vi "监测项目写入.vi"(8 "error in (no error)":errorcluster caption="错误输入（无错误）", 10 "字符串与值":cluster{"字符串":string, "值":u16}[](array[cluster]), 11 "SingleStepTestV3 输入":refnum<class "SingleStepTestV2.lvclass">) -> (0 "error out":errorcluster caption="错误输出", 3 "SingleStepTestV3 输出":refnum<class "SingleStepTestV2.lvclass">)   [LabVIEW 2022 SP3, in "SingleStepTestV2.lvlib" / "SingleStepTestV2.lvclass"]
uses:
  SingleStepTestV2.lvclass
  SingleStepTestV2.lvclass/SingleStepTestV2.ctl
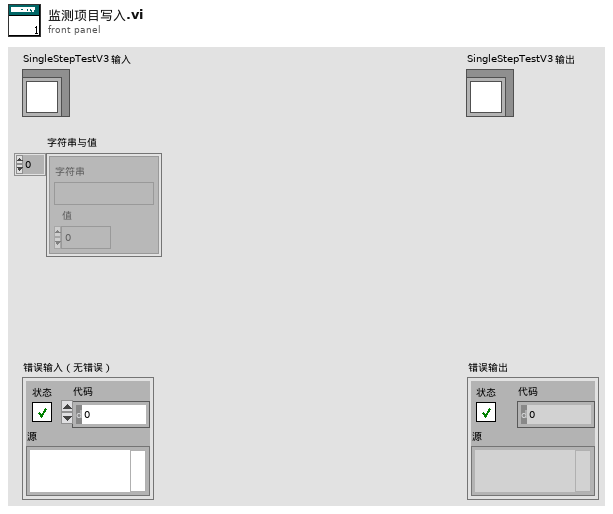
[diagram p1: front panel]
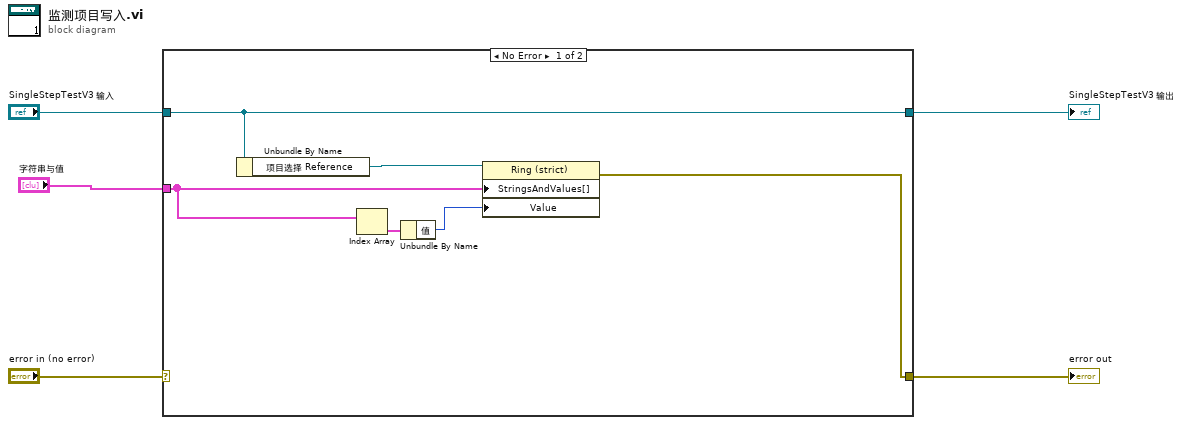
[diagram p0: block diagram]
diagram:
  n1 = case shown="No Error" "error in (no error)" {
    selector: "error in (no error)" -> [_ w13]
    tunnel: [w6 w13] -> w4
    tunnel: [w7 w12] -> w2
    tunnel: "SingleStepTestV3 输入" -> [w7 w12]
    tunnel: "字符串与值" -> [w11 _]
    frame No Error {
      n2 = Unbundle By Name(w7) -> ("项目选择 Reference"=w8:refnum<vi>)
      n3 = Index Array(array=w11) -> (element=w10:cluster{"字符串":string, "值":u16})  [unwired: 1 in]
      n4 = Unbundle By Name(w10) -> ("值"=w9:u16)
      n5 = property class="Ring (strict)"(reference=w8, "StringsAndValues[]"=w11, "Value"=w9) -> (error out=w6:errorcluster)  [unwired: 1 in, 1 out]
    }
    frame Error {
    }
  }
  "error out" <- w4
  "SingleStepTestV3 输出" <- w2
